vi "Write Settings Button.vi"(8 "error in (no error)":errorcluster, 10 "Settings Button":refnum<vi>, 11 "UI in":refnum<class "UI.lvclass">) -> (0 "error out":errorcluster, 3 "UI out":refnum<class "UI.lvclass">)   [LabVIEW 2015, in "Generic UI Actor.lvlib" / "UI.lvclass"]
uses:
  UI.lvclass
  UI.lvclass/UI.ctl
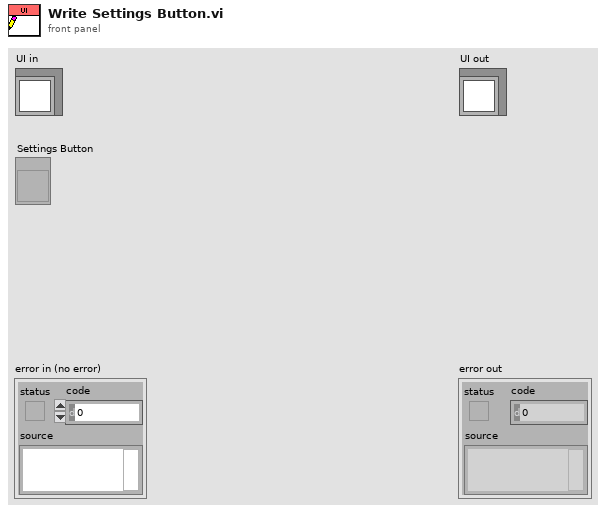
[diagram p1: front panel]
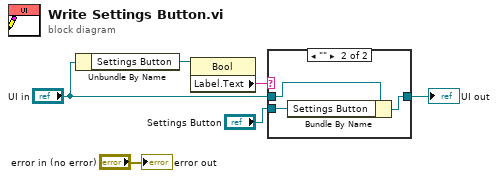
[diagram p0: block diagram]
diagram:
  n1 = Unbundle By Name("UI in") -> ("Settings Button"=w5:refnum<vi>)
  n2 = property class="Bool"(reference=w5) -> ("Label.Text"=w4:string)  [unwired: 1 in, 2 out]
  n3 = case shown="\"\"" w4 {
    tunnel: [w7 w9] -> w1
    tunnel: "UI in" -> [w7 w10]
    tunnel: "Settings Button" -> [_ w8]
    frame Default {
    }
    frame "" {
      n4 = Bundle By Name(cluster=w10, "Settings Button"=w8) -> (w9:refnum<class "UI.lvclass">)
    }
  }
  "UI out" <- w1
  "error out" <- "error in (no error)"
